vi "get piece from region 2.vi"   [LabVIEW 2018]
types:
  T1 = enum16{"shoulder", "elbow", "wrist", "base", "gripper"}
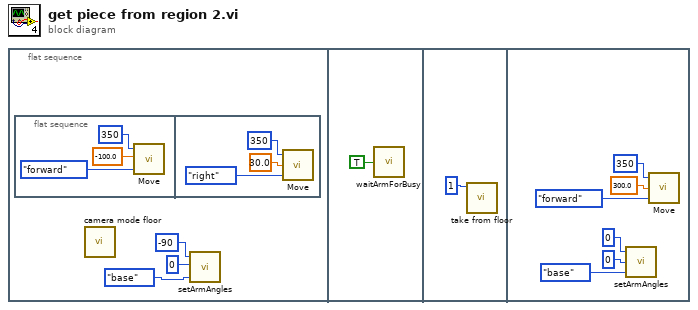
[diagram p0: block diagram]
diagram:
  n1 = flat-sequence {
    frame #0 {
      n2 = flat-sequence {
        frame #0 {
          n3 = call "Move.vi"("Enum"=enum16{"forward", "backward", "left", "right"}."forward", "distance"=-100.0, "speed"=350) -> ()  [unwired: 1 in]
        }
        frame #1 {
          n4 = call "Move.vi"("Enum"=enum16{"forward", "backward", "left", "right"}."right", "distance"=30.0, "speed"=350) -> ()  [unwired: 1 in]
        }
      }
      n5 = call "camera mode floor.vi"() -> ()  [unwired: 12 in]
      n6 = call "setArmAngles.vi"("Enum"=T1."base", "speed"=0, "angle"=-90) -> ()  [unwired: 1 in]
    }
    frame #1 {
      n7 = call "waitArmForBusy.vi"("base"=TRUE) -> ()
    }
    frame #2 {
      n8 = call "take from floor.vi"("m"=1) -> ()  [unwired: 11 in]
    }
    frame #3 {
      n9 = call "setArmAngles.vi"("Enum"=T1."base", "speed"=0, "angle"=0) -> ()  [unwired: 1 in]
      n10 = call "Move.vi"("Enum"=enum16{"forward", "backward", "left", "right"}."forward", "distance"=300.0, "speed"=350) -> ()  [unwired: 1 in]
    }
  }
